vi "ReadVXMCfg.vi"(8 "error in (no error)":errorcluster, 11 "VXMCfg in":refnum<class "VXMCfg.lvclass">) -> (0 "error out":errorcluster, 1 "VXM Properties.Serial Port 3":cluster{"Addr":string, "Enable":bool}, 2 "VXM Properties.Serial Port 2":cluster{"Addr":string, "Enable":bool}, 3 "VXMCfg out":refnum<class "VXMCfg.lvclass">, 5 "VXM Properties.Serial Port":cluster{"Addr":string, "Enable":bool})   [LabVIEW 2019, in "VXMCfg.lvclass"]
uses:
  VXMCfg.lvclass
  VXMCfg.lvclass/VXMCfg.ctl
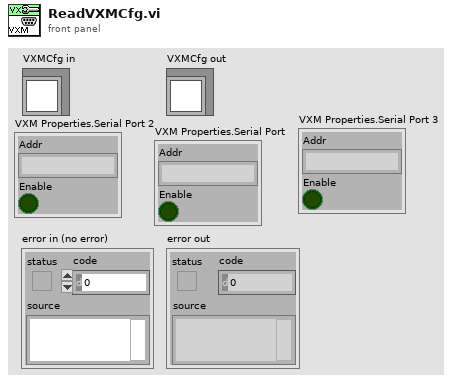
[diagram p1: front panel]
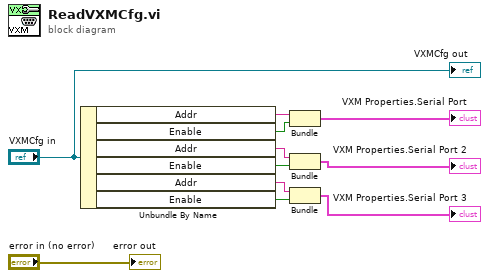
[diagram p0: block diagram]
diagram:
  n1 = Unbundle By Name("VXMCfg in") -> ("Addr"=w9:string, "Enable"=w8:bool, "Addr"=w7:string, "Enable"=w6:bool, "Addr"=w5:string, "Enable"=w4:bool)
  n2 = Bundle("Addr"=w9, "Enable"=w8) -> (→"VXM Properties.Serial Port":cluster{"Addr":string, "Enable":bool})  [unwired: 1 in]
  n3 = Bundle("Addr"=w7, "Enable"=w6) -> (→"VXM Properties.Serial Port 2":cluster{"Addr":string, "Enable":bool})  [unwired: 1 in]
  n4 = Bundle("Addr"=w5, "Enable"=w4) -> (→"VXM Properties.Serial Port 3":cluster{"Addr":string, "Enable":bool})  [unwired: 1 in]
  "error out" <- "error in (no error)"
  "VXMCfg out" <- "VXMCfg in"
